vi "Inherits from an Actor.vi"(7 "App Reference (this app)":refnum<vi>, 8 "error in (no error)":errorcluster, 11 "Path":path) -> (0 "error out":errorcluster, 1 "Default Actor Path":path, 2 "Is Path to Actor?":bool)   [LabVIEW 2020, in "Message Maker.lvlib"]
uses:
  Message Maker.lvlib
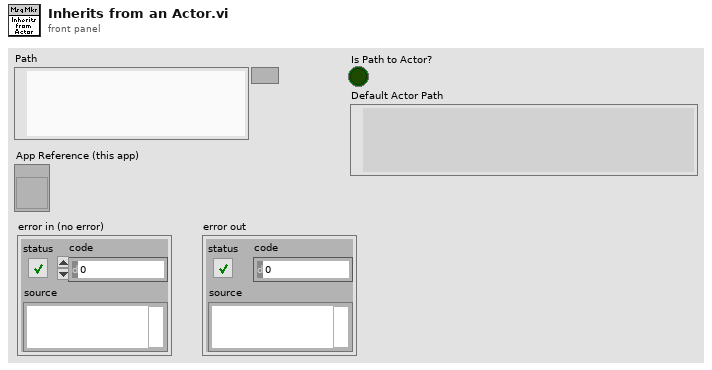
[diagram p1: front panel]
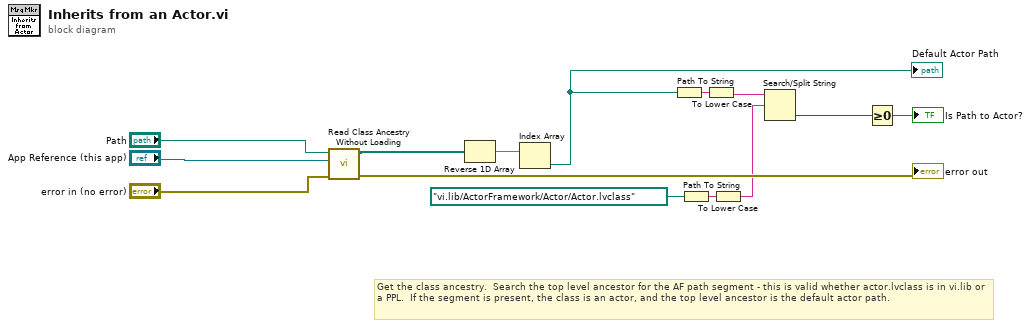
[diagram p0: block diagram]
diagram:
  # "Get the class ancestry.  Search the top level ancestor for the AF path segment - this is valid whether actor.lvclass is in vi.lib or a PPL.  If the segment is present, the class is an actor, and the top level ancestor is the default actor path."
  n1 = call <vilib>:"Read Class Ancestry Without Loading.vi"("error in (no error)"="error in (no error)", "App Reference (this app)"="App Reference (this app)", "LabVIEW Class Path"="Path") -> ("error out"=→"error out":errorcluster, "Class Ancestry"=w8:path[])  [unwired: 7 in]
  n2 = Reverse 1D Array(array=w8) -> (reversed array=w7:path[])
  n3 = Index Array(array=w7) -> (element=w9:path)  [unwired: 1 in]
  "Default Actor Path" <- w9
  n4 = Path To String(path=w9) -> (string=w5:string)
  n5 = Path To String(path=path "vi.lib/ActorFramework/Actor/Actor.lvclass") -> (string=w4:string)
  n6 = To Lower Case(string=w5) -> (all lower case string=w3:string)
  n7 = To Lower Case(string=w4) -> (all lower case string=w2:string)
  n8 = Search/Split String(string=w3, search string/char (-)=w2) -> (offset of match=w13:i32)  [unwired: 1 in, 2 out]
  n9 = Greater Or Equal To 0?(x=w13) -> (x >= 0?=→"Is Path to Actor?":bool)
